vi "Circus Root Path.vi"(8 "error in (no error)":errorcluster) -> (0 "error out":errorcluster, 3 "Circus Root Path":path)   [LabVIEW 2026, in "TALOS.lvlib"]
uses:
  TALOS.lvlib
  Global Memory.vi
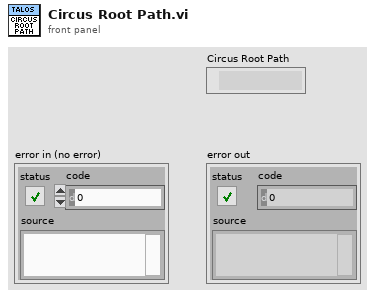
[diagram p1: front panel]
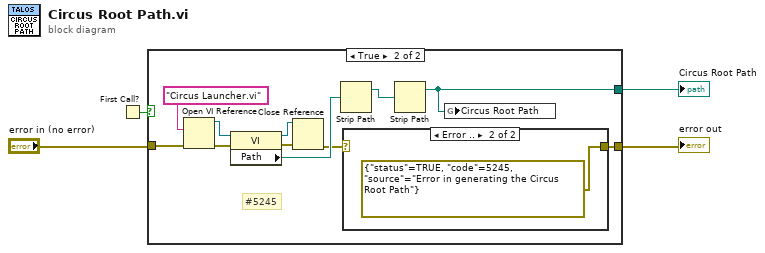
[diagram p0: block diagram]
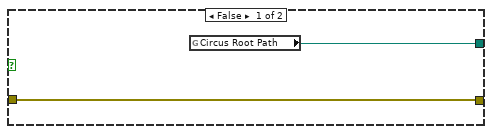
[diagram p2: hidden frame]
diagram:
  n1 = First Call?() -> (First Call?: T/F=w1:bool)
  n2 = case shown="True" w1 {
    tunnel: [w5 w9] -> w4
    tunnel: [w6 w7] -> w3
    tunnel: "error in (no error)" -> [w6 w17]
    frame False {
      n3 = global read "Global Memory.vi" "Circus Root Path"() -> (w5:path)
    }
    frame True {
      # "#5245"
      n4 = Open VI Reference(vi path="Circus Launcher.vi", error in (no error)=w17) -> (vi reference=w15:refnum<vi>, error out=w14:errorcluster)  [unwired: 4 in]
      n5 = property class="VI"(reference=w15, error in=w14) -> (reference out=w12:refnum<vi>, error out=w13:errorcluster, "Path"=w11:path)
      n6 = Close Reference(reference=w12, error in (no error)=w13) -> (error out=w8:errorcluster)
      n7 = Strip Path(path=w11) -> (stripped path=w10:path)  [unwired: 1 out]
      n8 = case shown="Error .." w8 {
        selector: w8 -> [w18 _]
        tunnel: [w18 errorcluster {"status"=TRUE, "code"=5245, "source"="Error in generating the Circus Root Path"} ("error IO")] -> w7
        frame No Error {
        }
        frame Error {
        }
      }
      n9 = Strip Path(path=w10) -> (stripped path=w9:path)  [unwired: 1 out]
      n10 = global write "Global Memory.vi" "Circus Root Path"(w9) -> ()
    }
  }
  "Circus Root Path" <- w4
  "error out" <- w3
